vi "Read Error.vi"() -> ()   [LabVIEW 2021, in "Mettler Toledo.lvlib"]
uses:
  Mettler Toledo.lvlib
  Controls/Settings Cluster.ctl
  <vilib>/regexp/Match Regular Expression.xnode
  support/Support Library.lvlib
  <vilib>/ptbypt/NI_PtbyPt.lvlib
panel:
  out "read buffer":string
  out "Connection Error":bool
  out "mass (g)":dbl
  out "Mettler Settings out":T1
  in  "Mettler Settings in":T1
  out "error out":errorcluster
  in  "error in (no error)":errorcluster
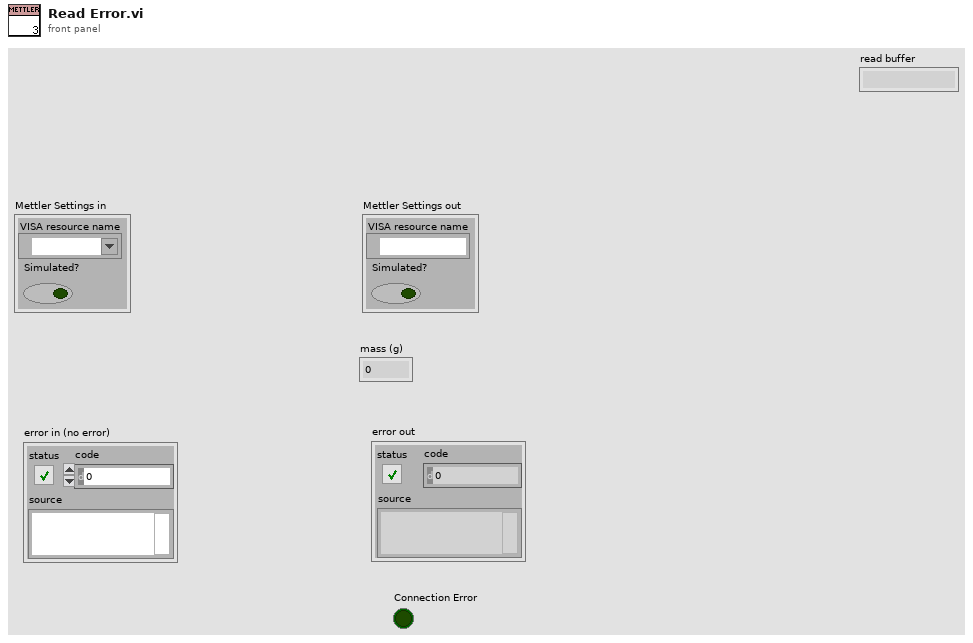
[diagram p1: front panel]
types:
  T1 = typedef "Mettler Toledo.lvlib/Settings Cluster.ctl" = cluster{"VISA resource name":refnum<visa-resource-name>, "Simulated?":bool}
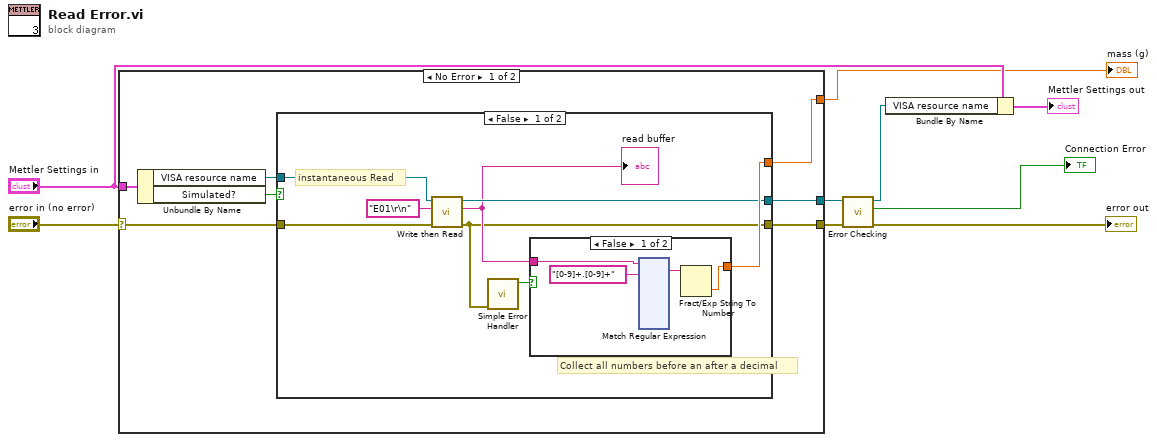
[diagram p0: block diagram]
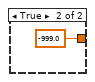
[diagram p2: hidden frame]
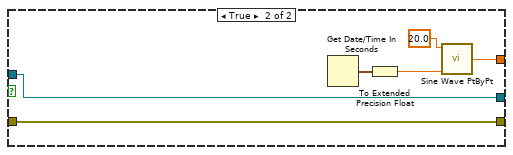
[diagram p3: hidden frame]
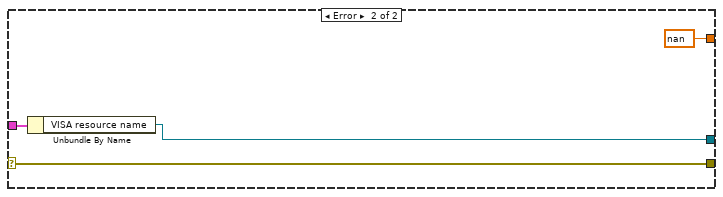
[diagram p4: hidden frame]
diagram:
  n1 = case shown="No Error" "error in (no error)" {
    selector: "error in (no error)" -> [w15 w161]
    tunnel: [w14 w161] -> w4
    tunnel: "Mettler Settings in" -> [w12 w159]
    tunnel: [w13 nan ("sine wave")] -> w7
    tunnel: [w10 w158] -> w5
    frame No Error {
      n2 = Unbundle By Name(w12) -> ("VISA resource name"=w11:refnum<visa-resource-name>, "Simulated?"=w16:bool)
      n3 = case shown="False" w16 {
        tunnel: [w17 w157] -> w14
        tunnel: w15 -> [w21 w157]
        tunnel: [w24 w153] -> w13
        tunnel: [w20 w152] -> w10
        tunnel: w11 -> [w23 w152]
        frame False {
          # "Collect all numbers before an after a decimal"
          # "instantaneous Read"
          n4 = call "Write then Read.vi"("error in"=w21, "write buffer"="E01\r\n" ("Command"), "VISA resource name in"=w23) -> ("error out"=w17:errorcluster, "read buffer"=w19:string, "VISA resource name out"=w20:refnum<visa-resource-name>)  [unwired: 5 in, 1 out]
          "read buffer" <- w19
          n5 = call <vilib>:"Simple Error Handler.vi"("error in (no error)"=w17) -> ("error?"=w18:bool)  [unwired: 4 in, 4 out]
          n6 = case shown="False" w18 {
            tunnel: w19 -> [w27 _]
            tunnel: [w25 -999.0] -> w24
            frame False {
              n7 = xnode "Match Regular Expression"("input string"=w27, "regular expression"="[0-9]+.[0-9]+" ("Regular Expression for Extracting Weight")) -> ("whole match"=w26:string)  [unwired: 4 in, 8 out]
              n8 = Fract/Exp String To Number(string=w26) -> (number=w25:dbl)  [unwired: 3 in, 1 out]
            }
            frame True {
            }
          }
        }
        frame True {
          n9 = Get Date/Time In Seconds() -> (seconds since 1Jan1904=w156:timestamp)
          n10 = To Extended Precision Float(1:w156) -> (0:w155:ext)
          n11 = call <vilib>:"Sine Wave PtByPt.vi"("time"=w155, "amplitude"=20.0) -> ("sine wave"=w153:dbl)  [unwired: 2 in]
        }
      }
    }
    frame Error {
      n12 = Unbundle By Name(w159) -> ("VISA resource name"=w158:refnum<visa-resource-name>)
    }
  }
  "mass (g)" <- w7
  n13 = call "Error Checking.vi"("error in (no error)"=w4, "VISA resource name"=w5) -> ("error out"=→"error out":errorcluster, "Connection Error"=→"Connection Error":bool, "VISA resource name"=w2:refnum<visa-resource-name>)  [unwired: 7 in]
  n14 = Bundle By Name(cluster="Mettler Settings in", "VISA resource name"=w2) -> (→"Mettler Settings out":T1)
